vi "SPADQ_ConfigSampRate.vi"(6 "mode":i32, 8 "error in (no error)":errorcluster, 9 "adq_num":i32, 10 "adq_cu_ptr in":refnum<k24>, 11 "ADQAPI Ref":refnum<k24>) -> (0 "error out":errorcluster, 1 "SampleRateHz":dbl, 2 "ADQ_MultiRecordSetup":u32, 3 "ADQAPI Ref (out)":refnum<k24>)   [LabVIEW 2022 SP3]
doc: "_____AlazarTech, Scope_____\n\nSet the Trigger delay"
uses:
  C:/Windows/System32/ADQAPI_dotNet_helper.dll
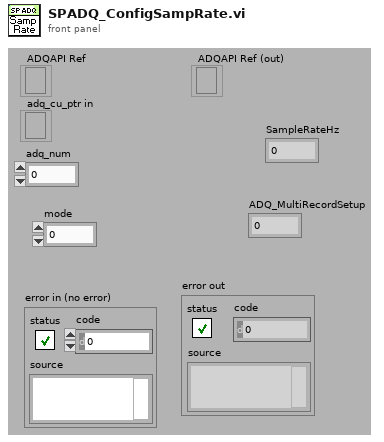
[diagram p1: front panel]
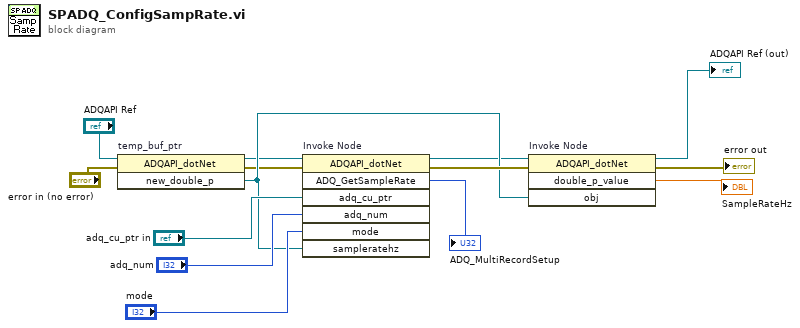
[diagram p0: block diagram]
diagram:
  n1 = invoke on="temp_buf_ptr" class="ADQAPI_dotNet" method="new_double_p"(reference="ADQAPI Ref", error in="error in (no error)") -> (reference out=w3:refnum<k24>, error out=w2:errorcluster, "new_double_p"=w9:refnum<k24>)  [unwired: 1 in]
  n2 = invoke on="Invoke Node" class="ADQAPI_dotNet" method="ADQ_GetSampleRate"(reference=w3, error in=w2, "adq_cu_ptr"="adq_cu_ptr in", "adq_num"="adq_num", "mode"="mode", "sampleratehz"=w9) -> (reference out=w8:refnum<k24>, error out=→"error out":errorcluster, "ADQ_GetSampleRate"=→"ADQ_MultiRecordSetup":i32)  [unwired: 1 in, 4 out]
  n3 = invoke on="Invoke Node" class="ADQAPI_dotNet" method="double_p_value"(reference=w8, "obj"=w9) -> (reference out=→"ADQAPI Ref (out)":refnum<k24>, "double_p_value"=→"SampleRateHz":dbl)  [unwired: 2 in, 2 out]
